vi "Dequeue FGV.vi"(8 "error in":errorcluster, 10 "Get Queue?":bool, 11 "queue in":refnum<queue>) -> (0 "error out":errorcluster, 1 "Message Data":variant, 2 "Message":string, 3 "queue out":refnum<queue>)   [LabVIEW 2020, in "State_Machine_Queue.lvlib"]
doc: "Dequeue FGV for the FGV queue based state machine.\n\n\n--------------------\nJuan Navarro\nLab It Studio"
uses:
  State_Machine_Queue.lvlib
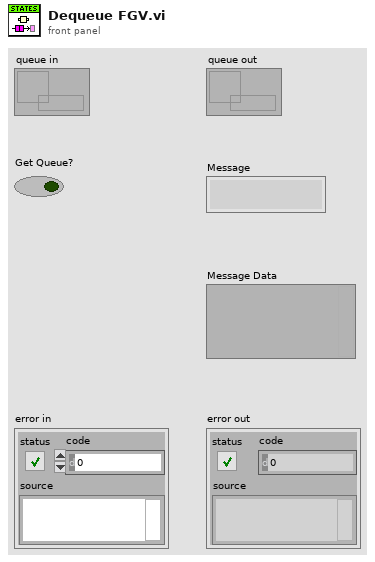
[diagram p1: front panel]
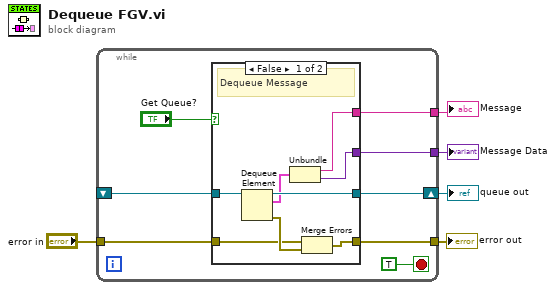
[diagram p0: block diagram]
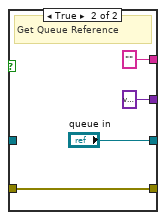
[diagram p2: hidden frame]
diagram:
  n1 = while {
    tunnel: "error in" -> [w12]
    tunnel: [w11] -> w2
    shift-right: [w10] -> w5
    shift-left: _ -> [w13]
    tunnel: [w8] -> w4
    tunnel: [w7] -> w3
    stop <- TRUE stop-if-true
    n2 = case shown="False" "Get Queue?" {
      tunnel: w13 -> [w21 _]
      tunnel: w12 -> [w15 w24]
      tunnel: [w14 w24] -> w11
      tunnel: [w20 "queue in"] -> w10
      tunnel: [w18 variant ("Variant")] -> w8
      tunnel: [w17 "" ("String")] -> w7
      frame False {
        # "Dequeue Message"
        n3 = Dequeue Element(queue=w21) -> (queue out=w20:refnum<queue>, element=w19:cluster{"State 2":string, "Data 2":variant}, error out=w16:errorcluster)  [unwired: 2 in, 1 out]
        n4 = Unbundle(w19) -> ("State 2"=w17:string, "Data 2"=w18:variant)
        n5 = Merge Errors(w15, w16) -> (w14:errorcluster)
      }
      frame True {
        # "Get Queue Reference"
      }
    }
  }
  "queue out" <- w5
  "Message Data" <- w4
  "Message" <- w3
  "error out" <- w2
